vi "NPC3SG Move Absolute.vi"(1 "Running":refnum<vi>, 3 "Drive New Abs. Positions":T1={"Drive X Set"=10.0, "Drive Y Set"=10.0, "Drive Z Set"=10.0} {"Drive X Set" min=10.0 max=160.0 step=0.1 format="%.3f"; "Drive Z Set" min=10.0 max=160.0 step=0.1 format="%.3f"; "Drive Y Set" min=10.0 max=160.0 step=0.1 format="%.3f"}, 4 "Drive Visa Name":refnum<visa-resource-name>="COM5") -> ()   [LabVIEW 2010]
uses:
  TypeDefs/NPC3SG Set Positions.ctl
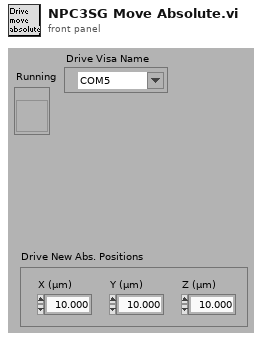
[diagram p1: front panel]
types:
  T1 = typedef "NPC3SG Set Positions.ctl" = cluster{"Drive X Set":dbl, "Drive Y Set":dbl, "Drive Z Set":dbl}
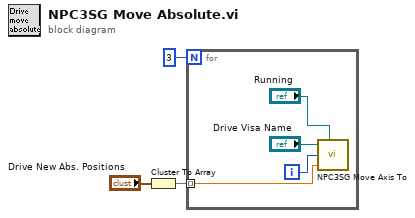
[diagram p0: block diagram]
diagram:
  n1 = Cluster To Array(cluster="Drive New Abs. Positions") -> (array=w1:dbl[])
  n2 = for {
    N: 3 -> [_]
    tunnel: w1 -> [w4] mode=indexing
    i -> [w6]
    n3 = call "NPC3SG Move Axis To.vi"("Drive Visa Name"="Drive Visa Name", "Running"="Running", "Axis"=w6, "Drive Set"=w4) -> ()  [unwired: 3 in, 1 out]
  }
